vi "Cal.vi"() -> ()   [LabVIEW 2010]
uses:
  C:/Program Files/National Instruments/LabVIEW 2010/examples/comm/dotnet/Calculator.dll
panel:
  out "multiply":dbl
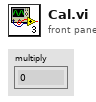
[diagram p1: front panel]
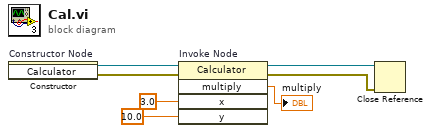
[diagram p0: block diagram]
diagram:
  n1 = constructor on="Constructor Node" class="Calculator"() -> (reference out=w7:refnum<k24>, error out=w6:errorcluster)  [unwired: 3 in, 1 out]
  n2 = invoke on="Invoke Node" class="Calculator" method="multiply"(reference=w7, error in=w6, "x"=3.0, "y"=10.0) -> (reference out=w4:refnum<k24>, error out=w5:errorcluster, "multiply"=→"multiply":dbl)  [unwired: 1 in, 2 out]
  n3 = Close Reference(reference=w4, error in (no error)=w5) -> ()  [unwired: 1 out]
